vi "Get Path to Read Only Console VI.vi"() -> (3 "Console VI Path":path)   [LabVIEW 2017, in "Communications Console Library.lvlib"]
uses:
  Communications Console Library.lvlib
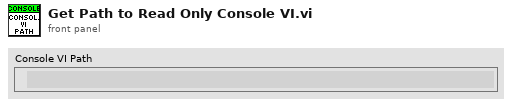
[diagram p1: front panel]
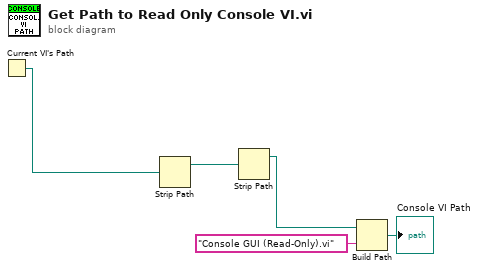
[diagram p0: block diagram]
diagram:
  n1 = Current VI's Path() -> (path=w5:path)
  n2 = Strip Path(path=w5) -> (stripped path=w4:path)  [unwired: 1 out]
  n3 = Strip Path(path=w4) -> (stripped path=w3:path)  [unwired: 1 out]
  n4 = Build Path(base path=w3, name or relative path="Console GUI (Read-Only).vi") -> (appended path=→"Console VI Path":path)
